vi "TRANSPOSE ARRAY.vi"() -> ()   [LabVIEW 2017]
panel:
  out "transposed array":dbl[][](array[numeric])
  out "Array":dbl[][](array[numeric])
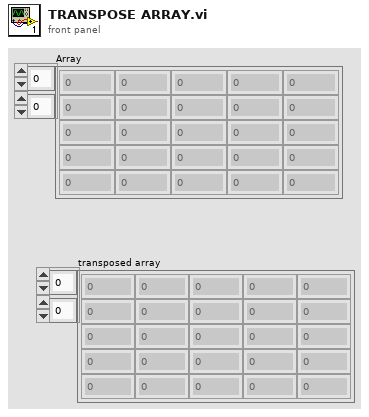
[diagram p1: front panel]
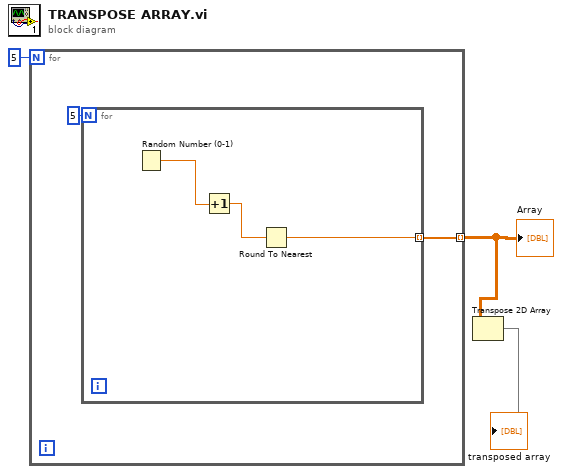
[diagram p0: block diagram]
diagram:
  n1 = for {
    N: 5 -> [_]
    tunnel: [w4] -> w2 mode=indexing
    n2 = for {
      N: 5 -> [_]
      tunnel: [w6] -> w4 mode=indexing
      n3 = Random Number (0-1)() -> (number: 0 to 1=w8:dbl)
      n4 = Increment(x=w8) -> (x+1=w7:dbl)
      n5 = Round To Nearest(number=w7) -> (nearest integer value=w6:dbl)
    }
  }
  "Array" <- w2
  n6 = Transpose 2D Array(2D array=w2) -> (transposed array=→"transposed array":dbl[][])
